vi "Phaco Ctrl.vi"() -> ()   [LabVIEW 2016]
uses:
  <vilib>/Platform/TimedLoop/XDataNode/timing_clust.ctl
  <vilib>/Platform/TimedLoop/XDataNode/nitl_modes.ctl
  <vilib>/Platform/TimedLoop/XDataNode/wakeup.ctl
  <vilib>/FPGAPlugInAG/PXI-7833R/niLvFpga_Open_PXI-7833R.vi
  <vilib>/Utility/error.llb/Error Cluster From Error Code.vi
  <vilib>/rvi/errors/niLvFpgaAdjustHostInterfaceError.vi
  <vilib>/FPGAPlugInAG/PXI-7833R/niLvFpga_Reset_PXI-7833R.vi
  <vilib>/FPGAPlugInAG/PXI-7833R/niLvFpga_Close_PXI-7833R.vi
  <vilib>/platform/TimedLoop/XDataNode/XDataNode.xnode
  <vilib>/rvi/interface/nirviOpenFPGA/nirviOpenFPGA.xnode
  FPGA Bitfiles/PhantomControlPI_FPGATarget_QuadCtr2_E2412E44.lvbitx
  IRISS_FPGA_IO.vi
  <vilib>/rvi/interface/nirviReadWriteControl/nirviReadWriteControl.xnode
  <vilib>/rvi/interface/nirviMethod/nirviMethod.xnode
  <vilib>/rvi/interface/nirviCloseFPGA/nirviCloseFPGA.xnode
  <vilib>/Platform/TimedLoop/XDataNode/XDNodeRunTimeDep.lvlib
  NiFpgaLv.dll
panel:
  in  "Max Limit [%]":dbl=600.0
  out "Ultrasound [%]":i32
  in  "Main Paddle":i8
  in  "Max Limit [mmHg]":dbl=600.0
  out "Boolean 2":bool
  out "Foot Paddle 3":dbl
  out "Ch A":dbl
  out "Ch B":dbl
  out "Paddle Reinit to Defualt":bool
  out "Vacuum Force\n[mmHg]":i32
  out "Waveform Chart":cluster{"f 2":dbl, "f":dbl}(graph)
  out "Error(s) Out on Program End":errorcluster
  in  "stop accurus":bool
  in  "stop prog":bool
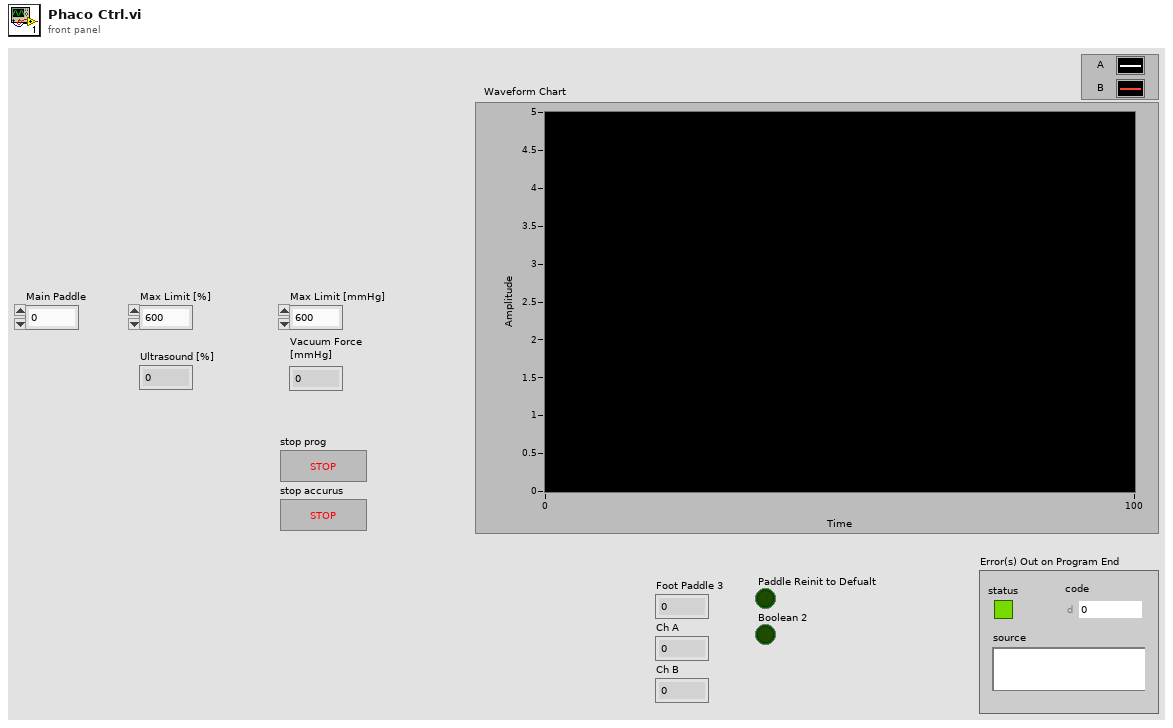
[diagram p1: front panel]
types:
  T1 = typedef "XDNodeRunTimeDep.lvlib/timing_clust.ctl" = cluster{"Expected End [f-1]":u64, "Actual End [f-1]":u64, "Finished Late? [f-1]":bool, "Expected End [i-1]":u64, "Actual End [i-1]":u64, "Finished Late? [i-1]":bool, "Expected Start [i]":u64, "Actual Start [i]":u64, "Expected Start [f]":u64, "Actual Start [f]":u64, "Source Name":string, "Structure Name":string, "Period":i64, "Deadline":i64, "Offset":i64, "Start":i64, "Priority":i32, "Timeout":i32, "Mode":T2, "Wakeup Reason":T3, "Error":errorcluster, "Source Type":string, "Secondary Source Type":string, "Global End Time":u64, "Global Start Time":u64, "Frame Duration":u64, "Iteration Duration":u64, "Assigned CPU":i32, "I/O Scan Engine Mode":u32}
  T2 = typedef "XDNodeRunTimeDep.lvlib/nitl_modes.ctl" = enum32{"No Change", "Process missed periods, maintain original phase", "Discard missed periods, maintain original phase", "Process missed periods, ignore original phase", "Discard missed periods, ignore original phase"}
  T3 = typedef "XDNodeRunTimeDep.lvlib/wakeup.ctl" = enum32{"Normal", "Aborted", "Asynchronous wakeup", "Timing source error", "Timed loop error", "Timeout"}
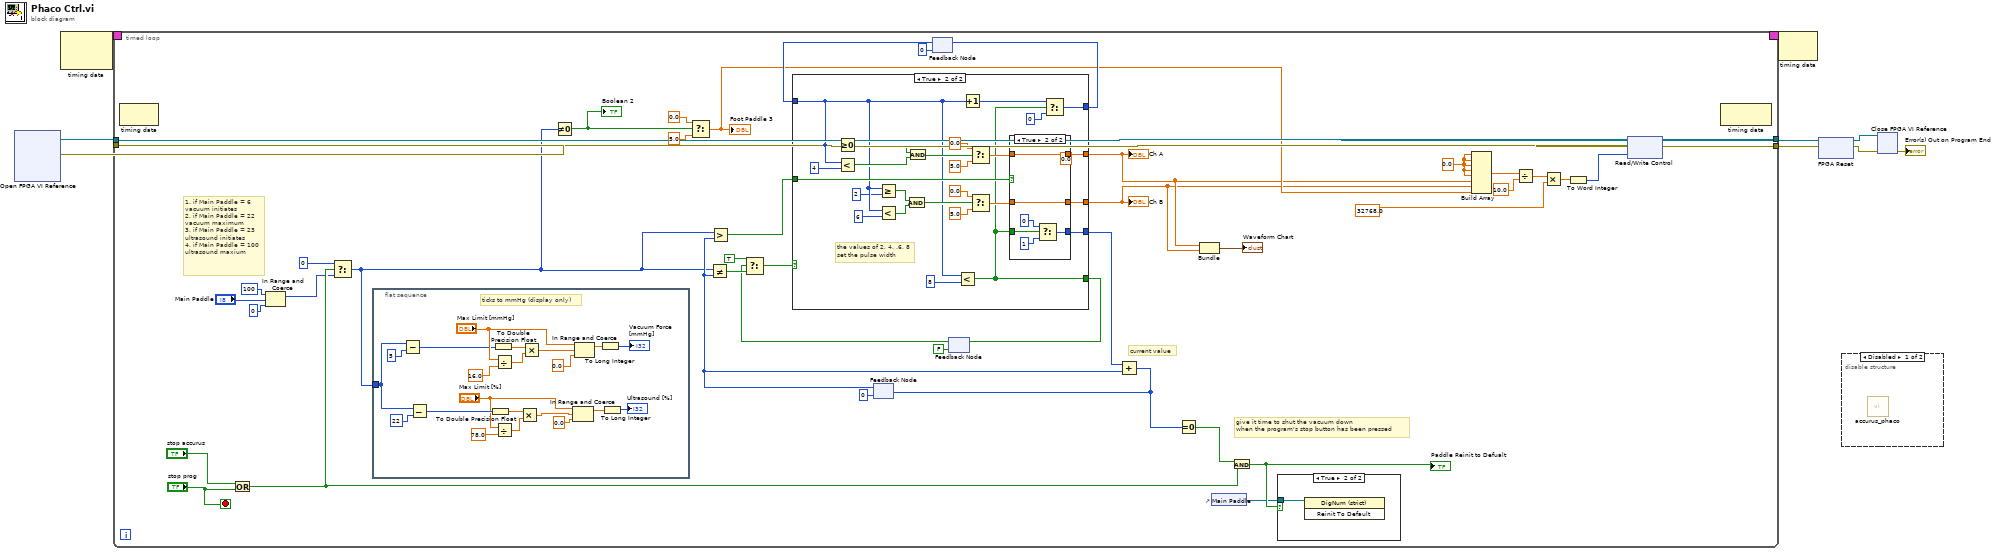
[diagram p0: block diagram]
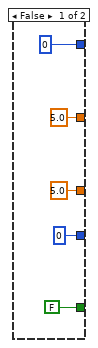
[diagram p4: hidden frame]
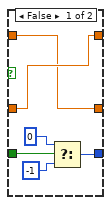
[diagram p5: hidden frame]
diagram:
  n1 = xnode "Open FPGA VI Reference"() -> ("FPGA VI Reference Out"=w7:refnum<k20>, "error out"=w6:errorcluster)  [unwired: 2 in]
  n2 = node-c288() -> (w9:T1)  [unwired: 2 in]
  n3 = timed-loop {
    timing: w9 -> [_]
    timing-out: [_] -> w8
    tunnel: w7 -> [w43]
    tunnel: w6 -> [w42]
    tunnel: [w45] -> w2
    tunnel: [w44] -> w1
    stop <- "stop prog" stop-if-true
    w21 = 0.0 ("element")
    (unwired) 0.0 ("element")
    # "1. if Main Paddle = 6\nvacuum initiates\n2. if Main Paddle = 22\nvacuum maximum\n3. if Main Paddle = 23\nultrasound initiates\n4. if Main Paddle = 100\nultrasound maxium"
    # "give it time to shut the vacuum down \nwhen the program's stop button has been pressed"
    # "current value"
    n4 = node-c288() -> ()  [unwired: 1 in, 1 out]
    n5 = Or(x="stop accurus", y="stop prog") -> (x .or. y?=w20:bool)
    n6 = In Range and Coerce(upper limit=i8 100, x="Main Paddle", lower limit=i8 0) -> (coerced(x)=w11:i8)  [unwired: 1 out]
    n7 = Select(t=i8 0, s=w20, f=w11) -> (s? t:f=w10:i8)
    n8 = flat-sequence {
      tunnel: w10 -> [w63]
      frame #0 {
        # "ticks to mmHg (display only)"
        n9 = Subtract(x=w63, y=i8 5) -> (x-y=w65:i8)
        n10 = Subtract(x=w63, y=i8 22) -> (x-y=w56:i8)
        n11 = To Double Precision Float(number=w56) -> (double precision float=w59:dbl)
        n12 = To Double Precision Float(number=w65) -> (double precision float=w74:dbl)
        n13 = Divide(x="Max Limit [mmHg]", y=16.0) -> (x/y=w69:dbl)
        n14 = Divide(x="Max Limit [%]", y=78.0) -> (x/y=w55:dbl)
        n15 = Multiply(x=w59, y=w55) -> (x*y=w58:dbl)
        n16 = Multiply(x=w74, y=w69) -> (x*y=w68:dbl)
        n17 = In Range and Coerce(upper limit="Max Limit [%]", x=w58, lower limit=0.0) -> (coerced(x)=w61:dbl)  [unwired: 1 out]
        n18 = In Range and Coerce(upper limit="Max Limit [mmHg]", x=w68, lower limit=0.0) -> (coerced(x)=w71:dbl)  [unwired: 1 out]
        n19 = To Long Integer(number=w71) -> (32bit integer=→"Vacuum Force\n[mmHg]":i32)
        n20 = To Long Integer(number=w61) -> (32bit integer=→"Ultrasound [%]":i32)
      }
    }
    n21 = Not Equal To 0?(x=w10) -> (x != 0?=w22:bool)
    "Boolean 2" <- w22
    n22 = Select(t=0.0, s=w22, f=5.0) -> (s? t:f=w19:dbl)
    "Foot Paddle 3" <- w19
    n23 = feedback #1(i8 0) -> (w29:i8)
    n24 = Not Equal?(x=w10, y=w29) -> (x != y?=w35:bool)
    n25 = Greater?(x=w10, y=w29) -> (0:w25:bool)
    n26 = feedback #2(i8 0) -> (w31:i8)
    n27 = feedback #3(FALSE) -> (w32:bool)
    n28 = Select(t=TRUE, s=w32, f=w35) -> (s? t:f=w34:bool)
    n29 = case shown="True" w34 {
      tunnel: [5.0 ("f") w93] -> w18
      tunnel: [5.0 ("f") w92] -> w17
      tunnel: [i8 0 ("f") w90] -> w28
      tunnel: [FALSE w85] -> w24
      tunnel: w25 -> [_ w91]
      tunnel: [i8 0 w87] -> w26
      tunnel: w31 -> [_ w89]
      frame False {
      }
      frame True {
        # "the values of 2, 4, ,6, 8 \nset the pulse width"
        n30 = Greater Or Equal To 0?(x=w89) -> (x >= 0?=w100:bool)
        n31 = Less?(x=w89, y=i8 4) -> (x < y?=w99:bool)
        n32 = Greater Or Equal?(x=w89, y=i8 2) -> (x >= y?=w98:bool)
        n33 = Less?(x=w89, y=i8 6) -> (x < y?=w97:bool)
        n34 = And(x=w98, y=w97) -> (x .and. y?=w96:bool)
        n35 = And(x=w100, y=w99) -> (x .and. y?=w101:bool)
        n36 = Less?(x=w89, y=i8 8) -> (x < y?=w85:bool)
        n37 = Increment(x=w89) -> (x+1=w88:i8)
        n38 = Select(t=0.0, s=w101, f=5.0) -> (s? t:f=w95:dbl)
        n39 = Select(t=0.0, s=w96, f=5.0) -> (s? t:f=w94:dbl)
        n40 = case shown="True" w91 {
          tunnel: w95 -> [w110 w116]
          tunnel: w94 -> [w111 w117]
          tunnel: [w110 w117] -> w92
          tunnel: [w111 w116] -> w93
          tunnel: w85 -> [w106 w115]
          tunnel: [w107 w114] -> w90
          frame False {
            n41 = Select(t=i8 0, s=w106, f=i8 -1) -> (s? t:f=w107:i8)
          }
          frame True {
            n42 = Select(t=i8 0, s=w115, f=i8 1) -> (s? t:f=w114:i8)
          }
        }
        n43 = Select(t=w88, s=w85, f=i8 0) -> (s? t:f=w87:i8)
      }
    }
    "Ch B" <- w17
    "Ch A" <- w18
    n44 = feedback-in #2(w26) -> ()
    n45 = feedback-in #3(w24) -> ()
    n46 = Add(x=w28, y=w29) -> (x+y=w39:i8)
    n47 = feedback-in #1(w39) -> ()
    n48 = Equal To 0?(x=w39) -> (x = 0?=w40:bool)
    n49 = Bundle("f"=w18, "f"=w17) -> (→"Waveform Chart":cluster{"f":dbl, "f":dbl})  [unwired: 1 in]
    n50 = control-ref of="Main Paddle"() -> (w15:refnum<vi>)
    n51 = And(x=w40, y=w20) -> (x .and. y?=w41:bool)
    "Paddle Reinit to Defualt" <- w41
    n52 = case shown="True" w41 {
      tunnel: w15 -> [_ w75]
      frame False {
      }
      frame True {
        n53 = invoke on="Invoke Node" class="DigNum (strict)" method="Reinit To Default"(reference=w75) -> ()  [unwired: 2 in, 3 out]
      }
    }
    n54 = Build Array(w21, w21, w21, w21, w21, w18, w17, w19) -> (w47:dbl[])
    n55 = Divide(x=w47, y=10.0) -> (x/y=w50:dbl[])
    n56 = Multiply(x=w50, y=32768.0) -> (x*y=w48:dbl[])
    n57 = To Word Integer(number=w48) -> (16bit integer=w46:i16[])
    n58 = xnode "Read/Write Control"("FPGA VI Reference In"=w43, "error in"=w42, "AO"=w46) -> ("FPGA VI Reference Out"=w45:refnum<k20>, "error out"=w44:errorcluster)
    n59 = node-c288() -> ()  [unwired: 1 in, 1 out]
  }
  n60 = node-c288(w8) -> ()  [unwired: 1 out]
  n61 = xnode "FPGA Reset"("FPGA VI Reference In"=w2, "error in"=w1) -> ("FPGA VI Reference Out"=w3:refnum<k20>, "error out"=w4:errorcluster)
  n62 = disable-structure shown="Disabled" {
    frame Disabled {
      n63 = call "accurus_phaco.vi"() -> ()  [unwired: 6 in, 6 out]
    }
    frame Enabled {
    }
  }
  n64 = xnode "Close FPGA VI Reference"("FPGA VI Reference In"=w3, "error in"=w4) -> ("error out"=→"Error(s) Out on Program End":errorcluster)
